vi "EXCESSdll.vi"(8 "error in (no error)":errorcluster, 11 "Inputs":cluster{"t":dbl, "p":dbl, "z":dbl[], "kph":i32}) -> (0 "error out":errorcluster, 3 "Outputs":T1)   [LabVIEW 2015]
doc: "subroutine EXCESSdll(t, p, z, kph, d, ve, ee, he, se, ae, ge, ierr, herr, herr_length)\n\nCompute excess properties as a function of temperature, pressure, and composition.\n\nINPUTS:\nt -- Temperature [K]\np -- Pressure [kPa]\nz -- Composition (array of mole fractions)\nkph -- Phase flag: 1 - Liquid 2 - Vapor 0 - Stable phase\n\nOUTPUTS:\nd -- Molar density [mol/L] (Send a negative density to the routine to use it as an initial guess.)\nve -- Excess volume [L/mol]\nee -- Excess energy [J/mol]\nhe -- Excess enthalpy [J/mol]\nse -- Excess entropy [J/mol-K]\nae -- Excess Helmholtz energy [J/mol]\nge -- Excess Gibbs energy [J/mol]\nierr -- Error flag: 0 - Successful\nherr -- Error string (character*255)\nherr_length -- length of variable herr (default: 255)"
uses:
  REFPROP.dll
panel:
  # "REFPROP-EXCESSdll.vi"
  # "void  EXCESSdll(double *t, double *p, double *z, int32_t *kph, double *d, double *ve, double *ee, double *he, double *se, double *ae, double *ge, int32_t *ierr, CStr herr, int32_t herr_length)"
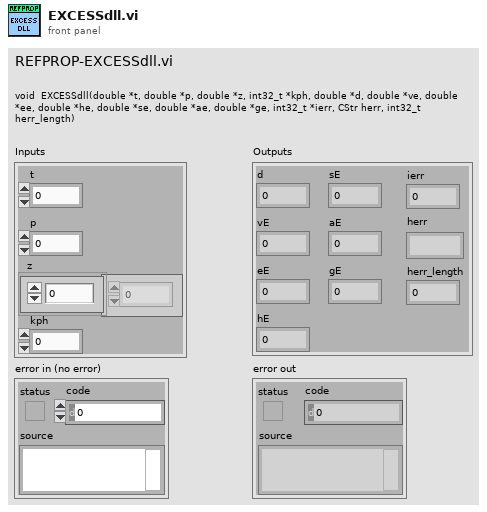
[diagram p1: front panel]
types:
  T1 = cluster{"d ":dbl, "vE ":dbl, "eE":dbl, "hE ":dbl, "sE ":dbl, "aE ":dbl, "gE ":dbl, "ierr ":i32, "herr ":string, "herr_length":i32}
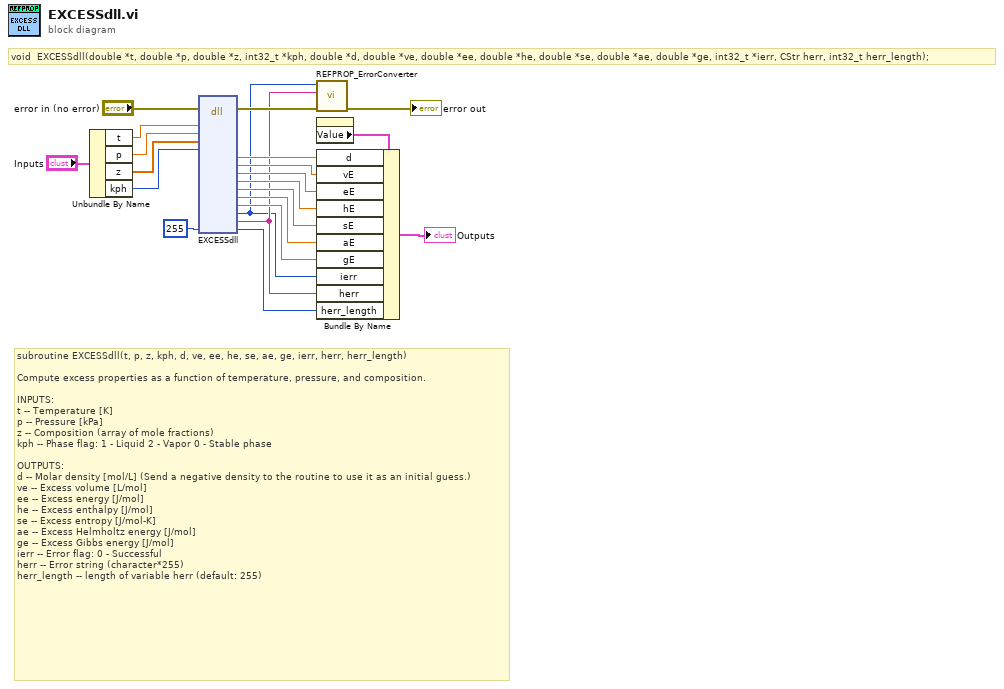
[diagram p0: block diagram]
diagram:
  # "void  EXCESSdll(double *t, double *p, double *z, int32_t *kph, double *d, double *ve, double *ee, double *he, double *se, double *ae, double *ge, int32_t *ierr, CStr herr, int32_t herr_length);"
  # "subroutine EXCESSdll(t, p, z, kph, d, ve, ee, he, se, ae, ge, ierr, herr, herr_length)\n\nCompute excess properties as a function of temperature, pressure, and composition.\n\nINPUTS:\nt -- Temperature [K]\np -- Pressure [kPa]\nz -- Composition (array of mole fractions)\nkph -- Phase flag: 1 - Liquid 2 - Vapor 0 - Stable phase\n\nOUTPUTS:\nd -- Molar density [mol/L] (Send a negative density to the routine to use it as an initial guess.)\nve -- Excess volume [L/mol]\nee -- Excess energy [J/mol]\nhe -- Excess enthalpy [J/mol]\nse -- Excess entropy [J/mol-K]\nae -- Excess Helmholtz energy [J/mol]\nge -- Excess Gibbs energy [J/mol]\nierr -- Error flag: 0 - Successful\nherr -- Error string (character*255)\nherr_length -- length of variable herr (default: 255)"
  n1 = Unbundle By Name("Inputs") -> ("t"=w15:dbl, "p"=w14:dbl, "z"=w13:dbl[], "kph"=w12:i32)
  n2 = dll-call lib="C:/Users/lauria/Desktop/REFPROP 10 LabVIEW Wrapper BETA/REFPROP/REFPROP.*" fn="EXCESSdll"(error in="error in (no error)", "t"=w15, "p"=w14, "z"=w13, "kph"=w12, "herr_length"=255 ("ln")) -> (error out=w20:errorcluster, "d"=w10:dbl, "ve"=w9:dbl, "ee"=w8:dbl, "he"=w7:dbl, "se"=w6:dbl, "ae"=w5:dbl, "ge"=w4:dbl, "ierr"=w1:i32, "herr"=w2:string, "herr_length"=w3:i32)  [unwired: 16 in, 1 out]
  n3 = call "REFPROP_ErrorConverter.vi"("error in (no error)"=w20, "Error Message"=w2, "Error Code"=w1) -> ("error out"=→"error out":errorcluster)  [unwired: 8 in]
  n4 = property on="Outputs" class="Clust (strict)"() -> ("Value"=w17:T1)  [unwired: 2 in, 2 out]
  n5 = Bundle By Name(cluster=w17, "d"=w10, "vE"=w9, "eE"=w8, "hE"=w7, "sE"=w6, "aE"=w5, "gE"=w4, "ierr"=w1, "herr"=w2, "herr_length"=w3) -> (→"Outputs":T1)
